vi "Opgave 4 Krig.vi"(11 "Antal runder":i32) -> (0 "Array med løbende Korttræk":u64[][](array[numeric]), 1 "Uafgjort":bool, 2 "Spiller B vinder 2":bool, 3 "Spiller A vinder":bool)   [LabVIEW 2019]
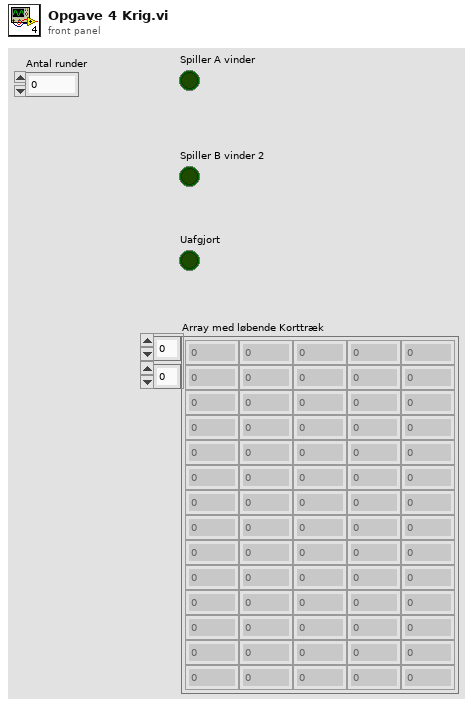
[diagram p1: front panel]
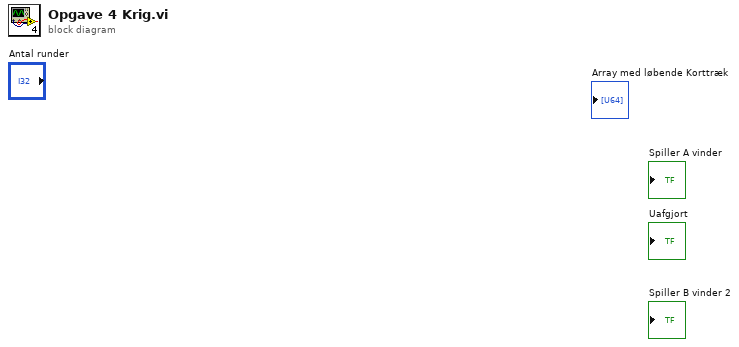
[diagram p0: block diagram]
diagram:
